vi "subFile Dialog.vi"(0 "start path":path, 1 "prompt":string, 3 "button label":string, 5 "selection mode":T1(ring), 7 "default name":string, 11 "error in":errorcluster, 12 "pattern (all files)":string, 14 "pattern label":string) -> (4 "selected path":path, 6 "selected paths":path[](array[path]), 8 "exists":bool, 10 "cancelled":bool, 15 "error out":errorcluster)   [LabVIEW 2026]
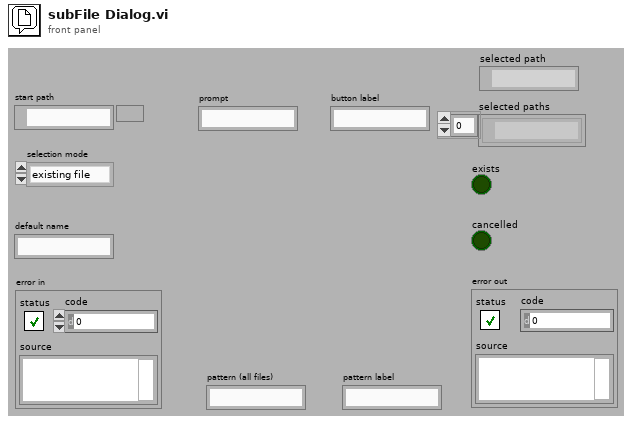
[diagram p1: front panel]
types:
  T1 = enum32{"existing file", "new file", "new or existing file", "existing dir", "new dir", "new or existing dir", "existing file (use LLBs)", "new file (use LLBs)", "new or existing file (use LLBs)", "new or existing file or directory (use LLBs)", "existing dir (use LLBs)", "new dir (use LLBs)", "new or existing dir (use LLBs)", "existing file or dir", "new file or dir", "new or existing file or dir", "existing file or dir (use LLBs)", "new file or dir (use LLBs)", "multi-select", "multi-select (use LLBs)"}
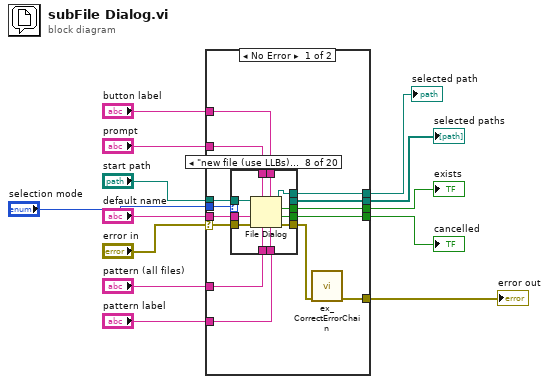
[diagram p0: block diagram]
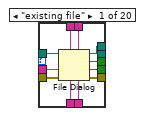
[diagram p2: hidden frame]
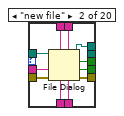
[diagram p3: hidden frame]
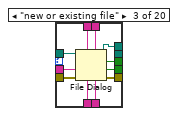
[diagram p4: hidden frame]
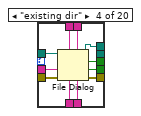
[diagram p5: hidden frame]
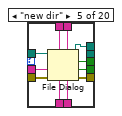
[diagram p6: hidden frame]
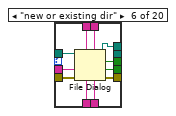
[diagram p7: hidden frame]
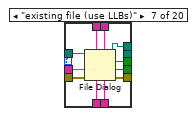
[diagram p8: hidden frame]
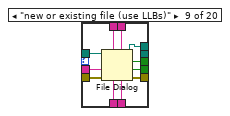
[diagram p9: hidden frame]
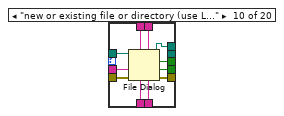
[diagram p10: hidden frame]
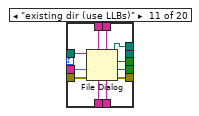
[diagram p11: hidden frame]
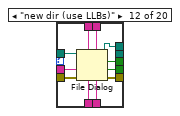
[diagram p12: hidden frame]
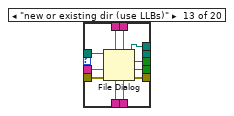
[diagram p13: hidden frame]
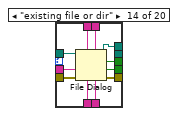
[diagram p14: hidden frame]
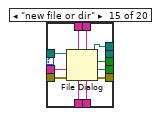
[diagram p15: hidden frame]
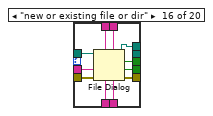
[diagram p16: hidden frame]
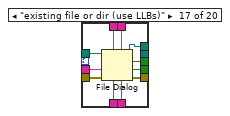
[diagram p17: hidden frame]
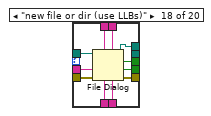
[diagram p18: hidden frame]
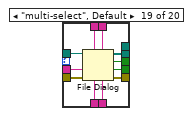
[diagram p19: hidden frame]
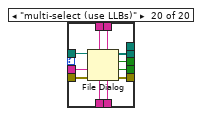
[diagram p20: hidden frame]
diagram:
  n1 = case shown="No Error" "error in" {
    selector: "error in" -> [w25 w248]
    tunnel: "start path" -> [w27 _]
    tunnel: "default name" -> [w26 _]
    tunnel: "pattern (all files)" -> [w24 _]
    tunnel: "prompt" -> [w23 _]
    tunnel: "button label" -> [w22 _]
    tunnel: "pattern label" -> [w21 _]
    tunnel: [w20 _] -> w6
    tunnel: [w19 _] -> w5
    tunnel: [w18 _] -> w4
    tunnel: [w17 _] -> w3
    tunnel: "selection mode" -> [w16 _]
    tunnel: [w14 w248] -> w1
    frame No Error {
      n2 = case shown="\"new file (use LLBs)\"" w16 {
        tunnel: w27 -> [w38 w49 w60 w71 w82 w93 w104 w115 w126 w137 w148 w159 w170 w181 w192 w203 w214 w225 w236 w247]
        tunnel: w26 -> [w37 w48 w59 w70 w81 w92 w103 w114 w125 w136 w147 w158 w169 w180 w191 w202 w213 w224 w235 w246]
        tunnel: w25 -> [w36 w47 w58 w69 w80 w91 w102 w113 w124 w135 w146 w157 w168 w179 w190 w201 w212 w223 w234 w245]
        tunnel: w24 -> [w35 w46 w57 w68 w79 w90 w101 w112 w123 w134 w145 w156 w167 w178 w189 w200 w211 w222 w233 w244]
        tunnel: w23 -> [w34 w45 w56 w67 w78 w89 w100 w111 w122 w133 w144 w155 w166 w177 w188 w199 w210 w221 w232 w243]
        tunnel: w22 -> [w33 w44 w55 w66 w77 w88 w99 w110 w121 w132 w143 w154 w165 w176 w187 w198 w209 w220 w231 w242]
        tunnel: w21 -> [w32 w43 w54 w65 w76 w87 w98 w109 w120 w131 w142 w153 w164 w175 w186 w197 w208 w219 w230 w241]
        tunnel: [_ _ _ _ _ _ _ _ _ _ _ _ _ _ _ _ _ _ w226 w237] -> w18
        tunnel: [w31 w42 w53 w64 w75 w86 w97 w108 w119 w130 w141 w152 w163 w174 w185 w196 w207 w218 w229 w240] -> w20
        tunnel: [w30 w41 w52 w63 w74 w85 w96 w107 w118 w129 w140 w151 w162 w173 w184 w195 w206 w217 w228 w239] -> w19
        tunnel: [w29 w40 w51 w62 w73 w84 w95 w106 w117 w128 w139 w150 w161 w172 w183 w194 w205 w216 w227 w238] -> w15
        tunnel: [w28 w39 w50 w61 w72 w83 w94 w105 w116 w127 w138 w149 w160 w171 w182 w193 w204 w215 _ _] -> w17
        frame "existing file" {
          n3 = File Dialog(4:w32, 5:w33, 6:w35, 7:w34, 8:w36, 9:w37, 11:w38) -> (0:w29:errorcluster, 1:w30:bool, 2:w31:bool, 3:w28:path)
        }
        frame "new file" {
          n4 = File Dialog(4:w43, 5:w44, 6:w46, 7:w45, 8:w47, 9:w48, 11:w49) -> (0:w40:errorcluster, 1:w41:bool, 2:w42:bool, 3:w39:path)
        }
        frame "new or existing file" {
          n5 = File Dialog(4:w54, 5:w55, 6:w57, 7:w56, 8:w58, 9:w59, 11:w60) -> (0:w51:errorcluster, 1:w52:bool, 2:w53:bool, 3:w50:path)
        }
        frame "existing dir" {
          n6 = File Dialog(4:w65, 5:w66, 6:w68, 7:w67, 8:w69, 9:w70, 11:w71) -> (0:w62:errorcluster, 1:w63:bool, 2:w64:bool, 3:w61:path)
        }
        frame "new dir" {
          n7 = File Dialog(4:w76, 5:w77, 6:w79, 7:w78, 8:w80, 9:w81, 11:w82) -> (0:w73:errorcluster, 1:w74:bool, 2:w75:bool, 3:w72:path)
        }
        frame "new or existing dir" {
          n8 = File Dialog(4:w87, 5:w88, 6:w90, 7:w89, 8:w91, 9:w92, 11:w93) -> (0:w84:errorcluster, 1:w85:bool, 2:w86:bool, 3:w83:path)
        }
        frame "existing file (use LLBs)" {
          n9 = File Dialog(4:w98, 5:w99, 6:w101, 7:w100, 8:w102, 9:w103, 11:w104) -> (0:w95:errorcluster, 1:w96:bool, 2:w97:bool, 3:w94:path)
        }
        frame "new file (use LLBs)" {
          n10 = File Dialog(4:w109, 5:w110, 6:w112, 7:w111, 8:w113, 9:w114, 11:w115) -> (0:w106:errorcluster, 1:w107:bool, 2:w108:bool, 3:w105:path)
        }
        frame "new or existing file (use LLBs)" {
          n11 = File Dialog(4:w120, 5:w121, 6:w123, 7:w122, 8:w124, 9:w125, 11:w126) -> (0:w117:errorcluster, 1:w118:bool, 2:w119:bool, 3:w116:path)
        }
        frame "new or existing file or directory (use LLBs)" {
          n12 = File Dialog(4:w131, 5:w132, 6:w134, 7:w133, 8:w135, 9:w136, 11:w137) -> (0:w128:errorcluster, 1:w129:bool, 2:w130:bool, 3:w127:path)
        }
        frame "existing dir (use LLBs)" {
          n13 = File Dialog(4:w142, 5:w143, 6:w145, 7:w144, 8:w146, 9:w147, 11:w148) -> (0:w139:errorcluster, 1:w140:bool, 2:w141:bool, 3:w138:path)
        }
        frame "new dir (use LLBs)" {
          n14 = File Dialog(4:w153, 5:w154, 6:w156, 7:w155, 8:w157, 9:w158, 11:w159) -> (0:w150:errorcluster, 1:w151:bool, 2:w152:bool, 3:w149:path)
        }
        frame "new or existing dir (use LLBs)" {
          n15 = File Dialog(4:w164, 5:w165, 6:w167, 7:w166, 8:w168, 9:w169, 11:w170) -> (0:w161:errorcluster, 1:w162:bool, 2:w163:bool, 3:w160:path)
        }
        frame "existing file or dir" {
          n16 = File Dialog(4:w175, 5:w176, 6:w178, 7:w177, 8:w179, 9:w180, 11:w181) -> (0:w172:errorcluster, 1:w173:bool, 2:w174:bool, 3:w171:path)
        }
        frame "new file or dir" {
          n17 = File Dialog(4:w186, 5:w187, 6:w189, 7:w188, 8:w190, 9:w191, 11:w192) -> (0:w183:errorcluster, 1:w184:bool, 2:w185:bool, 3:w182:path)
        }
        frame "new or existing file or dir" {
          n18 = File Dialog(4:w197, 5:w198, 6:w200, 7:w199, 8:w201, 9:w202, 11:w203) -> (0:w194:errorcluster, 1:w195:bool, 2:w196:bool, 3:w193:path)
        }
        frame "existing file or dir (use LLBs)" {
          n19 = File Dialog(4:w208, 5:w209, 6:w211, 7:w210, 8:w212, 9:w213, 11:w214) -> (0:w205:errorcluster, 1:w206:bool, 2:w207:bool, 3:w204:path)
        }
        frame "new file or dir (use LLBs)" {
          n20 = File Dialog(4:w219, 5:w220, 6:w222, 7:w221, 8:w223, 9:w224, 11:w225) -> (0:w216:errorcluster, 1:w217:bool, 2:w218:bool, 3:w215:path)
        }
        frame "multi-select", Default {
          n21 = File Dialog(4:w230, 5:w231, 6:w233, 7:w232, 8:w234, 9:w235, 11:w236) -> (0:w227:errorcluster, 1:w228:bool, 2:w229:bool, 3:w226:path[])
        }
        frame "multi-select (use LLBs)" {
          n22 = File Dialog(4:w241, 5:w242, 6:w244, 7:w243, 8:w245, 9:w246, 11:w247) -> (0:w238:errorcluster, 1:w239:bool, 2:w240:bool, 3:w237:path[])
        }
      }
      n23 = call "ex_CorrectErrorChain.vi"("error in (no error)"=w15) -> ("error out"=w14:errorcluster)  [unwired: 10 in]
    }
    frame Error {
    }
  }
  "exists" <- w6
  "cancelled" <- w5
  "error out" <- w1
  "selected paths" <- w4
  "selected path" <- w3
